vi "spectre status snmp .vi"(7 "Ring":u16(ring) items=["Get Status", "Get Info", "Get Uptime"], 8 "error in (no error)":errorcluster, 11 "IP Address":string="212.169.104.230") -> (0 "error out":errorcluster, 1 "Gateway Uptime":T1, 2 "Gateway Info":T2, 3 "Gateway Status":T3)   [LabVIEW 2017]
panel:
  out "Gateway supply voltage":waveform(dbl)(graph)
  out "Gateway temperature":waveform(u32)(graph)
  out "SnmpDataAsStrings":string[][](array[string])
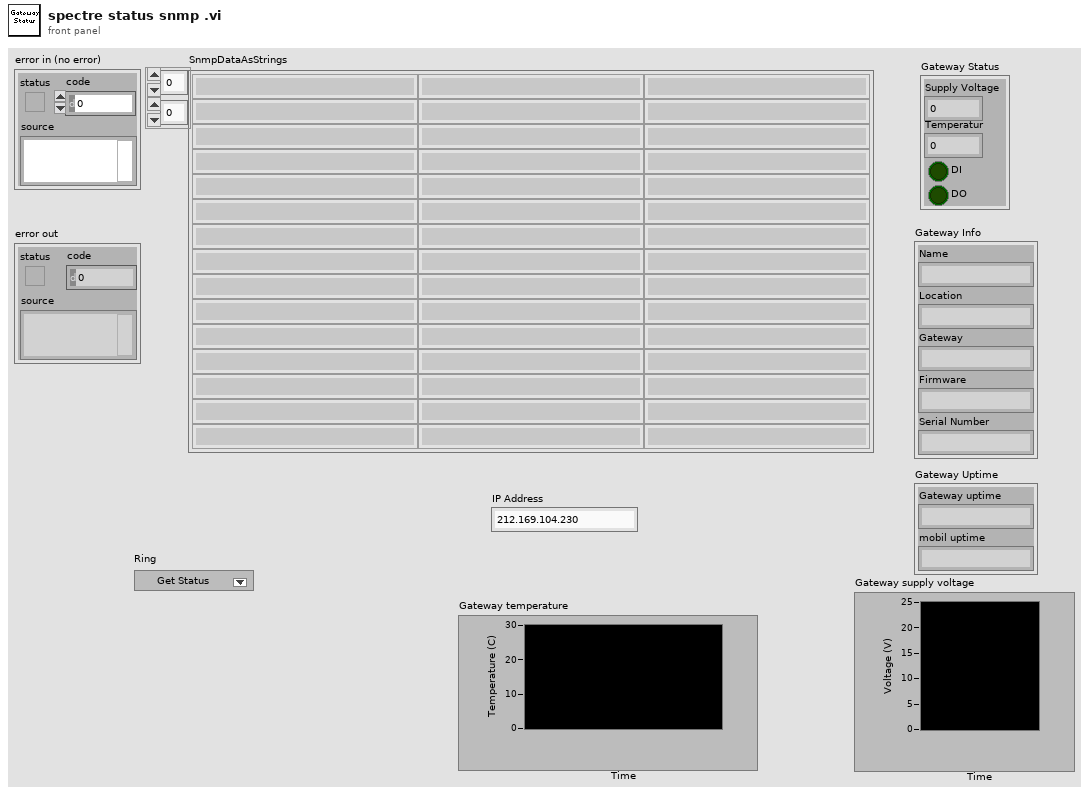
[diagram p1: front panel]
types:
  T1 = cluster{"Gateway uptime":string, "mobil uptime":string}
  T2 = cluster{"Name":string, "Location":string, "Gateway":string, "Firmware":string, "Serial Number":string}
  T3 = cluster{"Supply Voltage":dbl, "Temperatur":u32, "DI":bool, "DO":bool}
  T4 = cluster{"String":string, "String":string, "String":string, "String":string, "String":string}
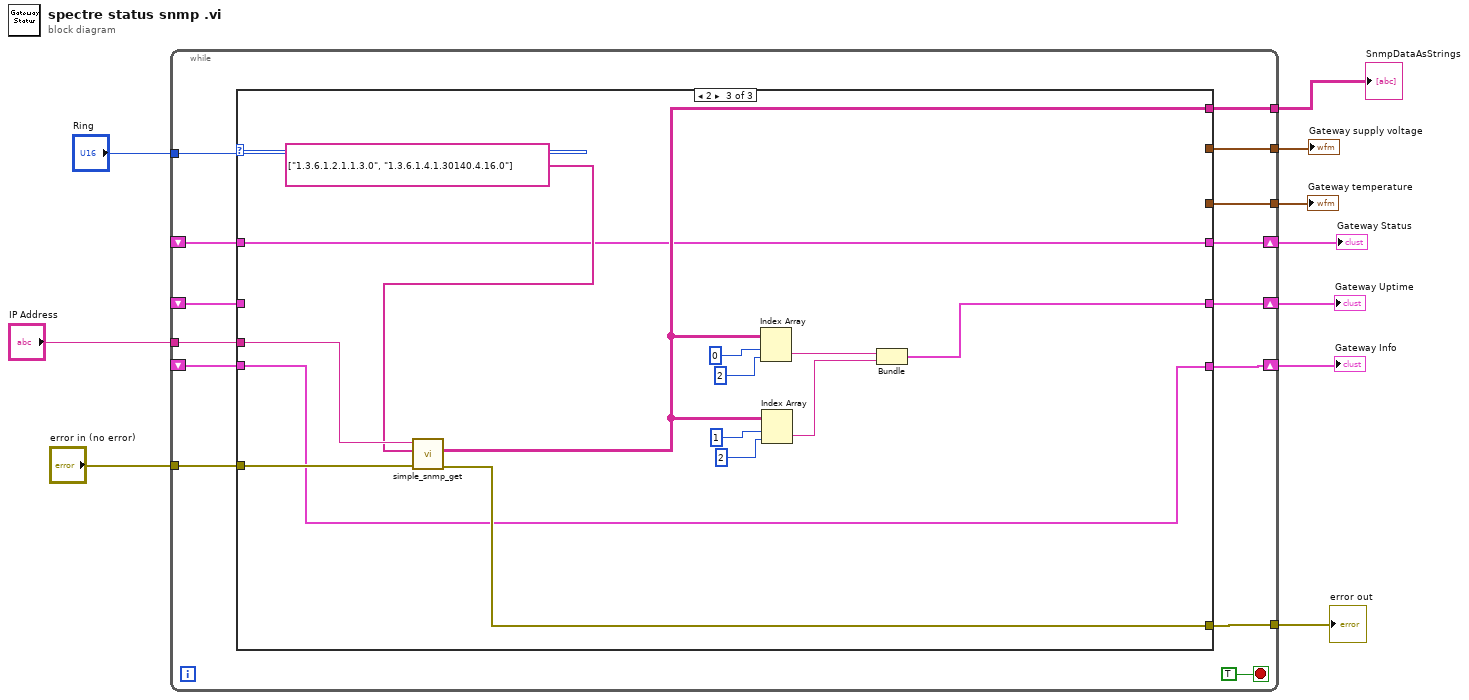
[diagram p0: block diagram]
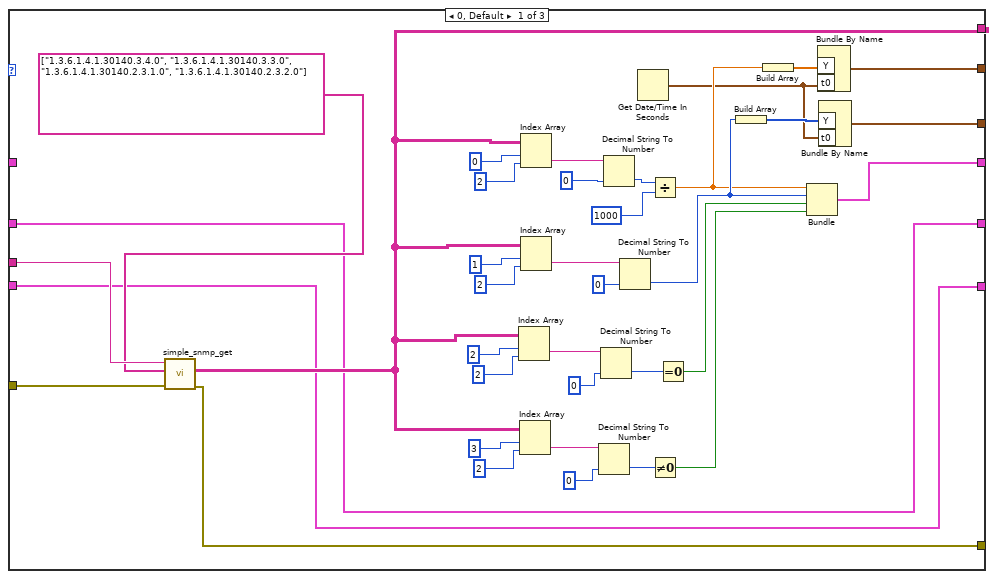
[diagram p2: hidden frame]
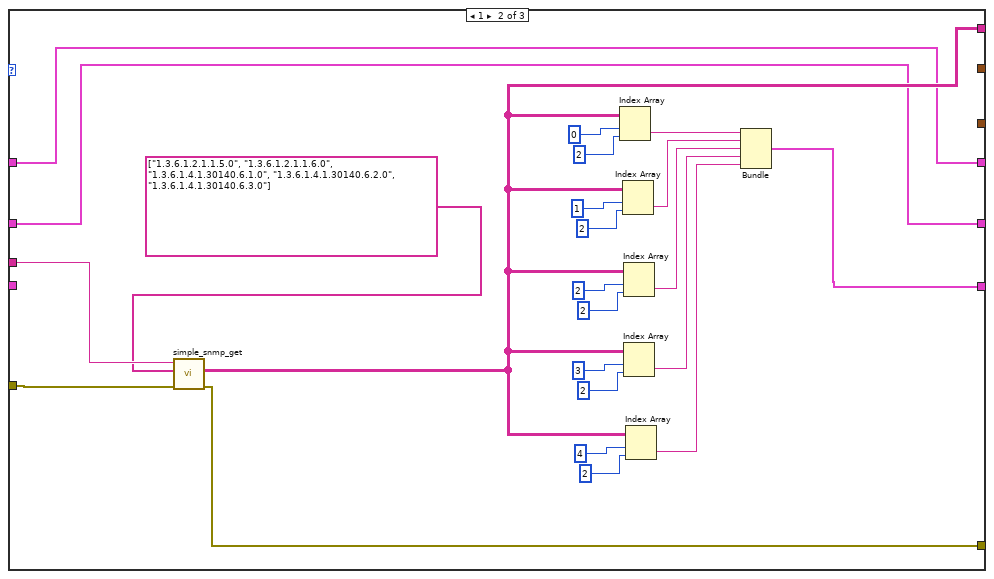
[diagram p3: hidden frame]
diagram:
  n1 = while {
    tunnel: "Ring" -> [w24]
    tunnel: "IP Address" -> [w23]
    tunnel: [w22] -> w8
    tunnel: [w21] -> w7
    tunnel: "error in (no error)" -> [w20]
    shift-right: [w18] -> w5
    shift-left: _ -> [w14]
    shift-right: [w17] -> w4
    shift-left: _ -> [w13]
    shift-right: [w16] -> w3
    shift-left: _ -> [w15]
    tunnel: [w12] -> w2
    tunnel: [w11] -> w1
    stop <- TRUE stop-if-true
    n2 = case shown="2" w24 {
      tunnel: w20 -> [w61 w84 w98]
      tunnel: w23 -> [w60 w83 w97]
      tunnel: [w36 w66 w96] -> w21
      tunnel: [w35 w65 w89] -> w22
      tunnel: [w33 w62 w87] -> w18
      tunnel: [w34 w63 w86] -> w17
      tunnel: [w32 w64 w85] -> w16
      tunnel: w15 -> [w32 _ w85]
      tunnel: w14 -> [w33 w62 _]
      tunnel: w13 -> [_ w63 w86]
      tunnel: [w27 _ _] -> w12
      tunnel: [w26 _ _] -> w11
      frame 0, Default {
        n3 = call "simple_snmp_get.vi"("error in (no error)"=w61, "OID Array"=string[] ["1.3.6.1.4.1.30140.3.4.0", "1.3.6.1.4.1.30140.3.3.0", "1.3.6.1.4.1.30140.2.3.1.0", "1.3.6.1.4.1.30140.2.3.2.0"], "IP Address of SNMP Device"=w60) -> ("error out"=w36:errorcluster, "SnmpDataAsStrings"=w35:string[][])  [unwired: 6 in, 1 out]
        n4 = Index Array(array=w35, index (row)=2, index (col)=2 ("disabled index (col)")) -> (element=w53:string)
        n5 = Index Array(array=w35, index (row)=3, index (col)=2 ("disabled index (col)")) -> (element=w55:string)
        n6 = Index Array(array=w35, index (row)=0, index (col)=2 ("disabled index (col)")) -> (element=w41:string)
        n7 = Index Array(array=w35, index (row)=1, index (col)=2 ("disabled index (col)")) -> (element=w47:string)
        n8 = Decimal String To Number(string=w55, default (0L)=u8 0 ("default (0 U32)")) -> (number=w57:u8)  [unwired: 1 in, 1 out]
        n9 = Decimal String To Number(string=w53, default (0L)=u8 0 ("default (0 U32)")) -> (number=w56:u8)  [unwired: 1 in, 1 out]
        n10 = Decimal String To Number(string=w41, default (0L)=u32 0 ("default (0 U32)")) -> (number=w43:u32)  [unwired: 1 in, 1 out]
        n11 = Decimal String To Number(string=w47, default (0L)=u32 0 ("default (0 U32)")) -> (number=w31:u32)  [unwired: 1 in, 1 out]
        n12 = Get Date/Time In Seconds() -> (seconds since 1Jan1904=w25:timestamp)
        n13 = Divide(x=w43, y=u16 1000) -> (x/y=w29:dbl)
        n14 = Not Equal To 0?(x=w57) -> (x != 0?=w59:bool)
        n15 = Equal To 0?(x=w56) -> (x = 0?=w58:bool)
        n16 = Build Array(w31) -> (w30:u32[])
        n17 = Build Array(w29) -> (w28:dbl[])
        n18 = Bundle(w29, w31, w58, w59) -> (w34:cluster{dbl, u32, bool, bool})  [unwired: 1 in]
        n19 = Bundle By Name("Y"=w28, "t0"=w25) -> (w27:waveform(dbl))  [unwired: 1 in]
        n20 = Bundle By Name("Y"=w30, "t0"=w25) -> (w26:waveform(u32))  [unwired: 1 in]
      }
      frame 1 {
        n21 = call "simple_snmp_get.vi"("error in (no error)"=w84, "OID Array"=string[] ["1.3.6.1.2.1.1.5.0", "1.3.6.1.2.1.1.6.0", "1.3.6.1.4.1.30140.6.1.0", "1.3.6.1.4.1.30140.6.2.0", "1.3.6.1.4.1.30140.6.3.0"], "IP Address of SNMP Device"=w83) -> ("error out"=w66:errorcluster, "SnmpDataAsStrings"=w65:string[][])  [unwired: 6 in, 1 out]
        n22 = Index Array(array=w65, index (row)=0, index (col)=2 ("disabled index (col)")) -> (element=w78:string)
        n23 = Index Array(array=w65, index (row)=1, index (col)=2 ("disabled index (col)")) -> (element=w79:string)
        n24 = Index Array(array=w65, index (row)=2, index (col)=2 ("disabled index (col)")) -> (element=w80:string)
        n25 = Index Array(array=w65, index (row)=3, index (col)=2 ("disabled index (col)")) -> (element=w81:string)
        n26 = Index Array(array=w65, index (row)=4, index (col)=2 ("disabled index (col)")) -> (element=w82:string)
        n27 = Bundle("String"=w78, "String"=w79, "String"=w80, "String"=w81, "String"=w82) -> (w64:T4)  [unwired: 1 in]
      }
      frame 2 {
        n28 = call "simple_snmp_get.vi"("error in (no error)"=w98, "OID Array"=string[] ["1.3.6.1.2.1.1.3.0", "1.3.6.1.4.1.30140.4.16.0"], "IP Address of SNMP Device"=w97) -> ("error out"=w96:errorcluster, "SnmpDataAsStrings"=w89:string[][])  [unwired: 6 in, 1 out]
        n29 = Index Array(array=w89, index (row)=0, index (col)=2 ("disabled index (col)")) -> (element=w94:string)
        n30 = Index Array(array=w89, index (row)=1, index (col)=2 ("disabled index (col)")) -> (element=w95:string)
        n31 = Bundle("String"=w94, "String"=w95) -> (w87:cluster{"String":string, "String":string})  [unwired: 1 in]
      }
    }
  }
  "SnmpDataAsStrings" <- w8
  "error out" <- w7
  "Gateway Uptime" <- w5
  "Gateway Status" <- w4
  "Gateway Info" <- w3
  "Gateway temperature" <- w1
  "Gateway supply voltage" <- w2
